vi "ObtieneDatosTabla.vi"(8 "error in (no error)":errorcluster, 11 "Prueba02 in":refnum<class "Prueba02.lvclass">) -> (0 "error out":errorcluster, 3 "Prueba02 out":refnum<class "Prueba02.lvclass">)   [LabVIEW 2019, in "Prueba02.lvclass"]
uses:
  Prueba02.lvclass
  Prueba02.lvclass/Prueba02.ctl
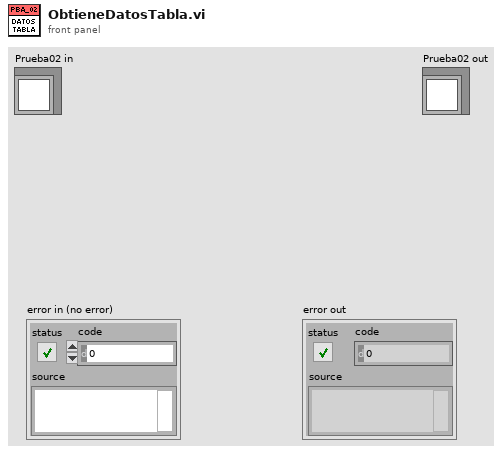
[diagram p1: front panel]
types:
  T1 = typedef "LVRowAndColumnTypeDef.ctl" = cluster{"Row":i32, "Column":i32}
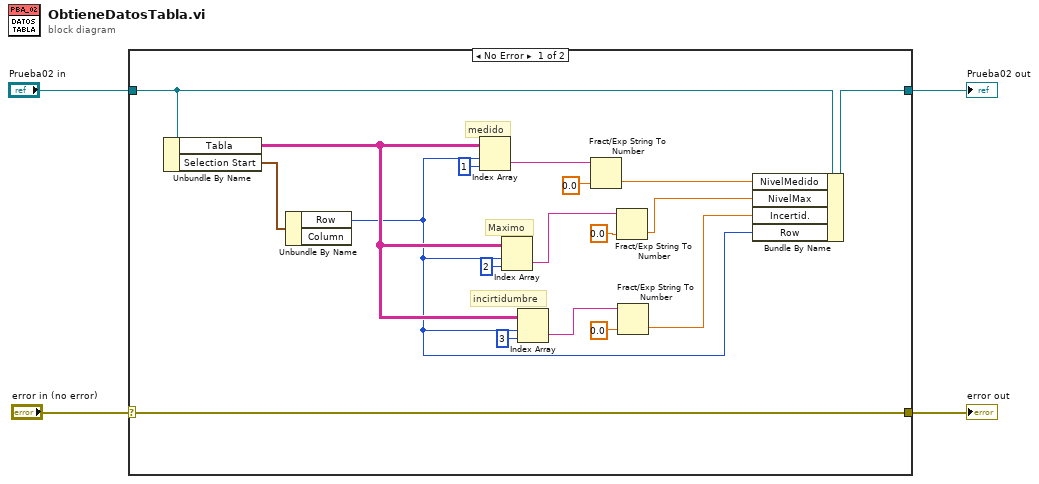
[diagram p0: block diagram]
diagram:
  n1 = case shown="No Error" "error in (no error)" {
    selector: "error in (no error)" -> [w12 w23]
    tunnel: [w22 w24] -> w4
    tunnel: "Prueba02 in" -> [w14 w24]
    tunnel: [w12 w23] -> w1
    frame No Error {
      # "incirtidumbre"
      # "Maximo"
      # "medido"
      n2 = Unbundle By Name(w14) -> ("Tabla"=w13:string[][], "Selection Start"=w6:T1)
      n3 = Unbundle By Name(w6) -> ("Row"=w5:i32)  [unwired: 1 out]
      n4 = Index Array(array=w13, index (row)=w5, index (col)=1 ("disabled index (col)")) -> (element=w21:string)
      n5 = Index Array(array=w13, index (row)=w5, index (col)=2 ("disabled index (col)")) -> (element=w15:string)
      n6 = Index Array(array=w13, index (row)=w5, index (col)=3 ("disabled index (col)")) -> (element=w16:string)
      n7 = Fract/Exp String To Number(string=w21, default (0 dbl)=0.0) -> (number=w20:dbl)  [unwired: 2 in, 1 out]
      n8 = Fract/Exp String To Number(string=w15, default (0 dbl)=0.0) -> (number=w9:dbl)  [unwired: 2 in, 1 out]
      n9 = Fract/Exp String To Number(string=w16, default (0 dbl)=0.0) -> (number=w8:dbl)  [unwired: 2 in, 1 out]
      n10 = Bundle By Name(cluster=w14, "NivelMedido"=w20, "NivelMax"=w9, "Incertid."=w8, "Row"=w5) -> (w22:refnum<class "Prueba02.lvclass">)
    }
    frame Error {
    }
  }
  "Prueba02 out" <- w4
  "error out" <- w1
